vi "Create All Message Queues.vi"(8 "error in (no error)":cluster{"状态":bool, "代码":i32, "源":string} caption="错误输入（无错误）") -> (0 "error out":cluster{"状态":bool, "代码":i32, "源":string} caption="错误输出", 3 "消息队列输出":T1)   [LabVIEW 2018, in "Message Queue.lvlib"]
doc: "本VI用于创建应用程序所需的所有消息队列。如应用程序需要两个以上消息队列，可右键单击上面的“消息队列”常量并选择“打开自定义类型”，将新的消息队列添加至该自定义类型，然后通过本VI进行初始化。"
uses:
  Message Queue.lvlib
  All Message Queues.ctl
  Message Cluster.ctl
  Enqueue Message (Single).vi
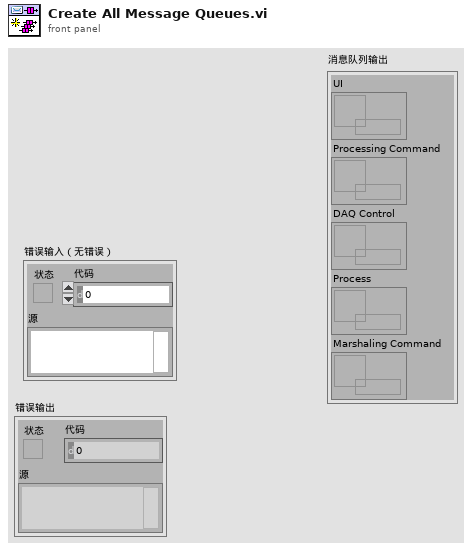
[diagram p1: front panel]
types:
  T1 = typedef "Message Queue.lvlib/All Message Queues.ctl" = cluster{"UI Updata":refnum<queue>, "Processing Command":refnum<queue>, "DAQ Control":refnum<queue>, "Camera Control":refnum<queue>, "Marshaling Command":refnum<queue>}
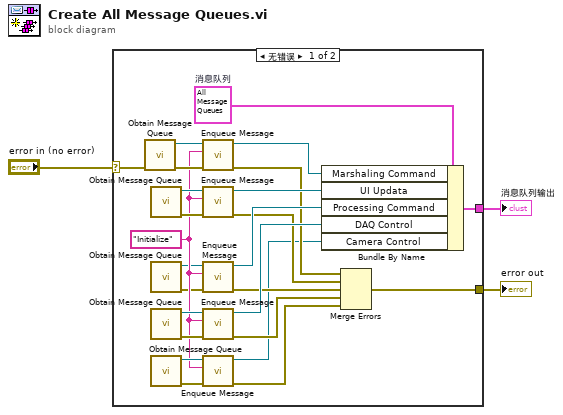
[diagram p0: block diagram]
diagram:
  n1 = case shown="无错误" "error in (no error)" {
    selector: "error in (no error)" -> [w26 w29]
    tunnel: [w14 w29] -> w3
    tunnel: [w27 _] -> w2
    frame No Error {
      w8 = "Initialize" ("Message")
      w28 = T1 {"UI Updata"=refnum, "Processing Command"=refnum, "DAQ Control"=refnum, "Camera Control"=refnum, "Marshaling Command"=refnum}  # 消息队列
      n2 = call "Obtain Message Queue.vi"("error in (no error)"=w26) -> ("error out"=w25:cluster{"状态":bool, "代码":i32, "源":string}, "消息队列"=w24:refnum<queue>)  [unwired: 9 in]
      n3 = call "Obtain Message Queue.vi"() -> ("error out"=w23:cluster{"状态":bool, "代码":i32, "源":string}, "消息队列"=w22:refnum<queue>)  [unwired: 10 in]
      n4 = call "Obtain Message Queue.vi"() -> ("error out"=w4:cluster{"状态":bool, "代码":i32, "源":string}, "消息队列"=w5:refnum<queue>)  [unwired: 10 in]
      n5 = call "Obtain Message Queue.vi"() -> ("error out"=w21:cluster{"状态":bool, "代码":i32, "源":string}, "消息队列"=w20:refnum<queue>)  [unwired: 10 in]
      n6 = call "Obtain Message Queue.vi"() -> ("error out"=w10:cluster{"状态":bool, "代码":i32, "源":string}, "消息队列"=w9:refnum<queue>)  [unwired: 10 in]
      n7 = call-poly "Enqueue Message.vi"("error in (no error)"=w25, "消息"=w8, "消息队列"=w24) -> ("error out"=w15:cluster{"状态":bool, "代码":i32, "源":string}, "消息队列副本"=w19:refnum<queue>)  [unwired: 7 in]
      n8 = call-poly "Enqueue Message.vi"("error in (no error)"=w23, "消息"=w8, "消息队列"=w22) -> ("error out"=w13:cluster{"状态":bool, "代码":i32, "源":string}, "消息队列副本"=w18:refnum<queue>)  [unwired: 7 in]
      n9 = call-poly "Enqueue Message.vi"("error in (no error)"=w4, "消息"=w8, "消息队列"=w5) -> ("error out"=w12:cluster{"状态":bool, "代码":i32, "源":string}, "消息队列副本"=w17:refnum<queue>)  [unwired: 7 in]
      n10 = call-poly "Enqueue Message.vi"("error in (no error)"=w21, "消息"=w8, "消息队列"=w20) -> ("error out"=w11:cluster{"状态":bool, "代码":i32, "源":string}, "消息队列副本"=w16:refnum<queue>)  [unwired: 7 in]
      n11 = call-poly "Enqueue Message.vi"("error in (no error)"=w10, "消息"=w8, "消息队列"=w9) -> ("error out"=w6:cluster{"状态":bool, "代码":i32, "源":string}, "消息队列副本"=w7:refnum<queue>)  [unwired: 7 in]
      n12 = Bundle By Name(cluster=w28, "Marshaling Command"=w19, "UI Updata"=w18, "Processing Command"=w17, "DAQ Control"=w16, "Camera Control"=w7) -> (w27:T1)
      n13 = Merge Errors(w15, w13, w12, w11, w6) -> (w14:errorcluster)
    }
    frame Error {
    }
  }
  "消息队列输出" <- w2
  "error out" <- w3
